vi "Erase Message.vi"(8 "error in (no error)":errorcluster, 11 "Channel GUI in":refnum<class "Channel GUI.lvclass">) -> (0 "error out":errorcluster, 3 "Channel GUI out":refnum<class "Channel GUI.lvclass">)   [LabVIEW 2018, in "Channel GUI.lvclass"]
uses:
  Channel GUI.lvclass
  Channel GUI.lvclass/Channel GUI.ctl
  Stream/Stream.lvclass
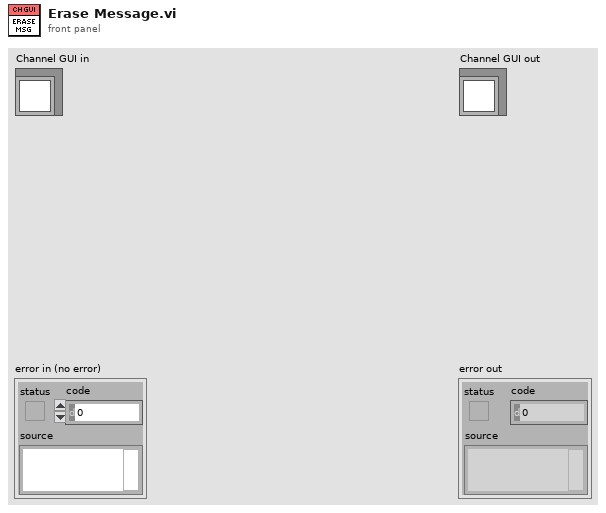
[diagram p1: front panel]
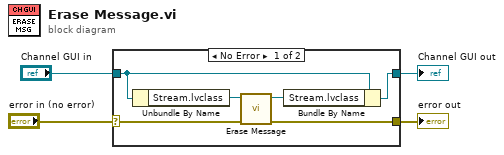
[diagram p0: block diagram]
diagram:
  n1 = case shown="No Error" "error in (no error)" {
    selector: "error in (no error)" -> [w7 w12]
    tunnel: [w8 w12] -> w3
    tunnel: [w9 w11] -> w1
    tunnel: "Channel GUI in" -> [w10 w11]
    frame No Error {
      n2 = Unbundle By Name(w10) -> ("Stream.lvclass"=w6:refnum<class "Stream.lvclass">)
      n3 = call "Erase Message.vi"("error in (no error)"=w7, "Stream in"=w6) -> ("error out"=w8:errorcluster, "Stream out"=w5:refnum<class "Stream.lvclass">)  [unwired: 8 in]
      n4 = Bundle By Name(cluster=w10, "Stream.lvclass"=w5) -> (w9:refnum<class "Channel GUI.lvclass">)
    }
    frame Error {
    }
  }
  "error out" <- w3
  "Channel GUI out" <- w1
